vi "Shutdown.vi"(8 "error in":errorcluster, 11 "Report in":refnum<class "Report.lvclass">) -> (0 "error out":errorcluster, 3 "Report out":refnum<class "Report.lvclass">)   [LabVIEW 2023, in "Report.lvlib" / "Report.lvclass"]
uses:
  Report.lvclass
  Report.lvclass/Report.ctl
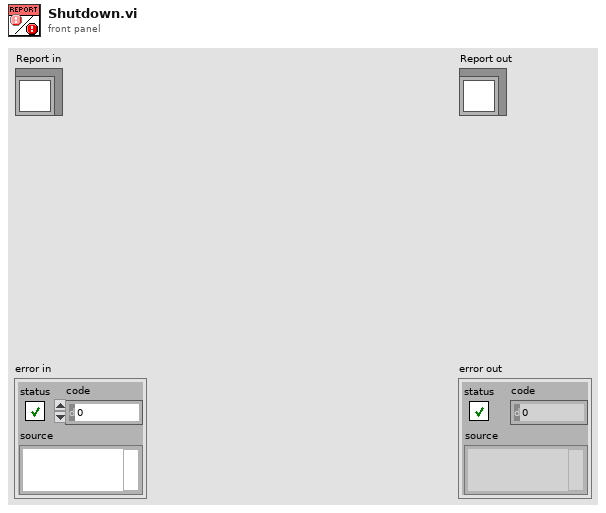
[diagram p1: front panel]
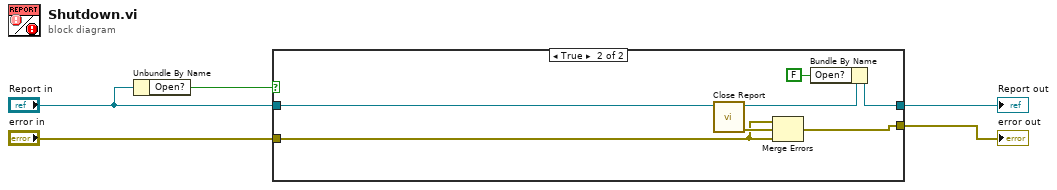
[diagram p0: block diagram]
diagram:
  n1 = Unbundle By Name("Report in") -> ("Open?"=w1:bool)
  n2 = case shown="True" w1 {
    tunnel: [w7 w9] -> w5
    tunnel: "error in" -> [w6 w10]
    tunnel: [w6 w12] -> w3
    tunnel: "Report in" -> [w7 w11]
    frame False {
    }
    frame True {
      n3 = call-dynamic "Close Report.vi"("Report in"=w11) -> ("error out"=w13:errorcluster, "Report out"=w14:refnum<class "Report.lvclass">)  [unwired: 9 in]
      n4 = Merge Errors(w10, w13, w10) -> (w12:errorcluster)
      n5 = Bundle By Name(cluster=w14, "Open?"=FALSE) -> (w9:refnum<class "Report.lvclass">)
    }
  }
  "error out" <- w3
  "Report out" <- w5
